vi "Add Attribute - Null.vi"(8 "error in (no error)":errorcluster, 10 "Attribute":string, 11 "YAML Parser in":refnum<class "YAML Parser.lvclass">) -> (0 "error out":errorcluster, 3 "YAML Parser out":refnum<class "YAML Parser.lvclass">)   [LabVIEW 2015, in "YAML Parser.lvclass"]
uses:
  YAML Parser.lvclass
  YAML Parser.lvclass/YAML Parser.ctl
panel:
  out "replaced":bool
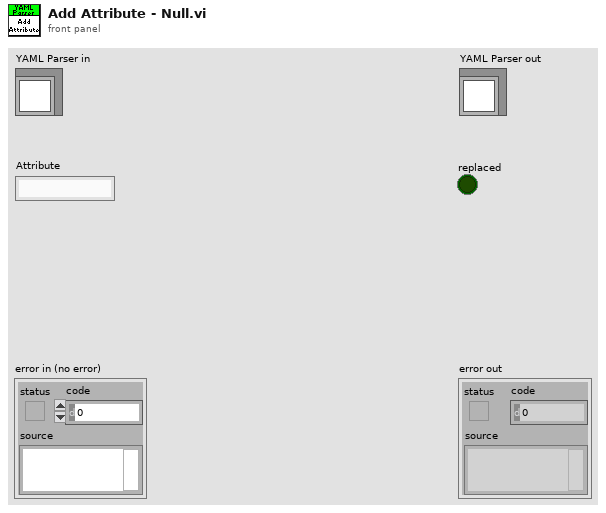
[diagram p1: front panel]
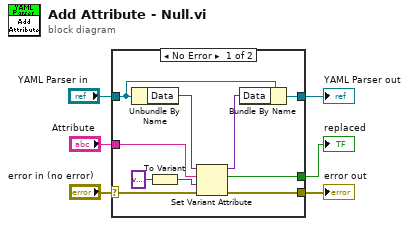
[diagram p0: block diagram]
diagram:
  n1 = case shown="No Error" "error in (no error)" {
    selector: "error in (no error)" -> [w14 w18]
    tunnel: [w13 w18] -> w5
    tunnel: [w16 w17] -> w3
    tunnel: "YAML Parser in" -> [w15 w17]
    tunnel: "Attribute" -> [w10 _]
    tunnel: [w9 _] -> w1
    frame No Error {
      n2 = Unbundle By Name(w15) -> ("Data"=w12:variant)
      n3 = To Variant(anything=variant) -> (Variant=w7:variant)
      n4 = Set Variant Attribute(Variant=w12, name=w10, value=w7, error in=w14) -> (Variant out=w11:variant, replaced=w9:bool, error out=w13:errorcluster)
      n5 = Bundle By Name(cluster=w15, "Data"=w11) -> (w16:refnum<class "YAML Parser.lvclass">)
    }
    frame Error {
    }
  }
  "error out" <- w5
  "YAML Parser out" <- w3
  "replaced" <- w1
